vi "Initialization VI.vi"(8 "error in (no error)":errorcluster, 10 "Custom XML":string, 11 "Device Item Ref in":T1 format="%.0x") -> (0 "error out":errorcluster, 3 "Device Item Ref out":T1 format="%.0x")   [LabVIEW 2016, in "UDP Sender System Explorer.lvlib"]
uses:
  <vilib>/NI Veristand/Custom Device API/Custom Device Item Ref.ctl
  UDP Sender System Explorer.lvlib
  <vilib>/NI Veristand/Custom Device API/Custom Device API.lvlib
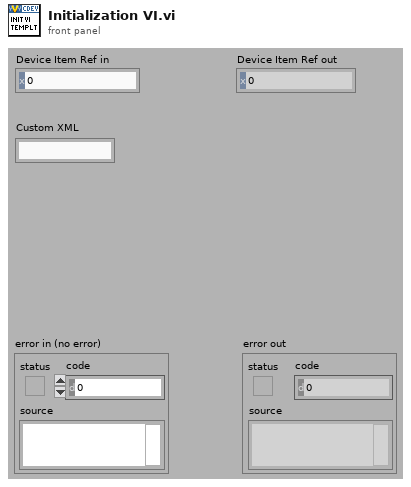
[diagram p1: front panel]
types:
  T1 = typedef "Custom Device API.lvlib/Custom Device Item Ref.ctl" = u64
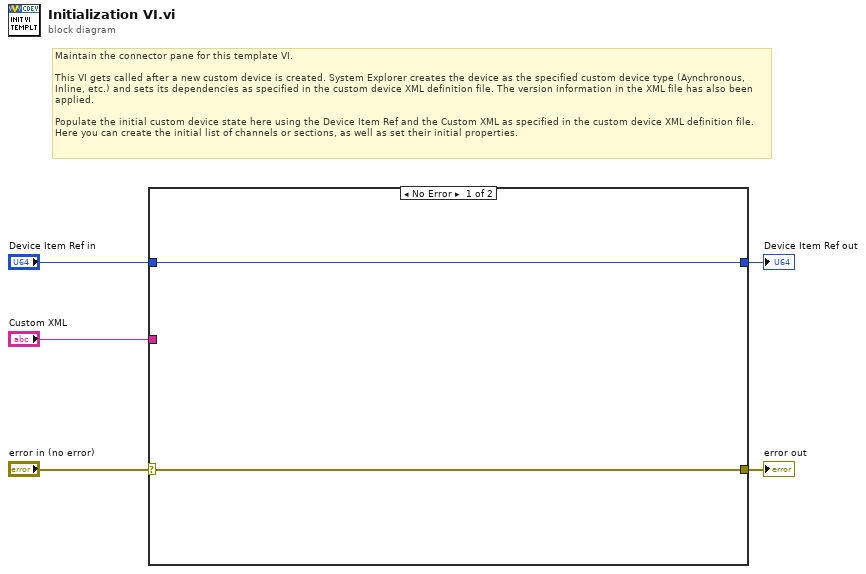
[diagram p0: block diagram]
diagram:
  # "Maintain the connector pane for this template VI.\n\nThis VI gets called after a new custom device is created. System Explorer creates the device as the specified custom device type (Aynchronous, Inline, etc.) and sets its dependencies as specified in the custom device XML definition file. The version information in the XML file has also been applied.\n\nPopulate the initial custom device state here using the Device Item Ref and the Custom XML as specified in the custom device XML definition file. Here you can create the initial list of channels or sections, as well as set their initial properties."
  n1 = case shown="No Error" "error in (no error)" {
    selector: "error in (no error)" -> [w6 w9]
    tunnel: [w6 w9] -> w5
    tunnel: [w7 w8] -> w3
    tunnel: "Device Item Ref in" -> [w7 w8]
    tunnel: "Custom XML" -> [_ _]
    frame No Error {
    }
    frame Error {
    }
  }
  "error out" <- w5
  "Device Item Ref out" <- w3
